vi "GetBdcst.vi"(8 "ErrorArray":errorcluster[](array[cluster]), 10 "BdcstInfo":variant, 11 "TestBase.lvclass":refnum<class "TestBase.lvclass">) -> (0 "ErrorArray":errorcluster[](array[cluster]), 3 "TestBase.lvclass":refnum<class "TestBase.lvclass">)   [LabVIEW 2014, in "TestBase.lvclass"]
uses:
  TestBase.lvclass
  TypeDefs/BdcstInfo.ctl
  TestBase.lvclass/TestBase.ctl
  WfrmGenerator/WfrmModule/Protected/Broadcasts/clBroadcastEvents.ctl
  WfrmGenerator/WfrmModule/Protected/clEventType.ctl
  Sampler/SamplerModule/Protected/Broadcasts/clBroadcastEvents.ctl
  Sampler/SamplerModule/Protected/clEventType.ctl
  FunctionGenerator/FGenModule/Protected/Broadcasts/clBroadcastEvents.ctl
  FunctionGenerator/FGenModule/Protected/clEventType.ctl
  Sync/SyncModule/Protected/Broadcasts/clBroadcastEvents.ctl
  Sync/SyncModule/Protected/clEventType.ctl
  Accessors/Read ErrorSeverity.vi
  <vilib>/Utility/error.llb/Error Cluster From Error Code.vi
  <vilib>/ErrorRing/Error Ring.xnode
  <userlib>/NIST/NISTErrorLib/NISTErrorLib.lvlib
  WfrmGenerator/WfrmModule/WfrmModule.lvlib
  Sync/SyncModule/SyncModule.lvlib
  Sampler/SamplerModule/SamplerModule.lvlib
  FunctionGenerator/FGenModule/FGenModule.lvlib
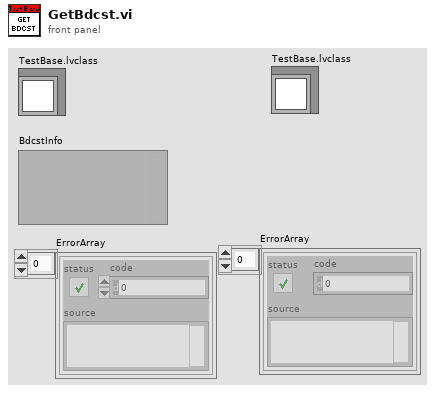
[diagram p1: front panel]
types:
  T1 = typedef "TestBase.lvclass/BdcstInfo.ctl" = cluster{"ModuleID":i32, "ModuleType":enum16{"Wfrm", "FGen", "Sampler", "Sync", "Analysis", "Sensor"}, "UserEvtRef":variant, "ScriptCmd":string}
  T2 = enum16{"Wfrm", "FGen", "Sampler", "Sync", "Analysis", "Sensor"}
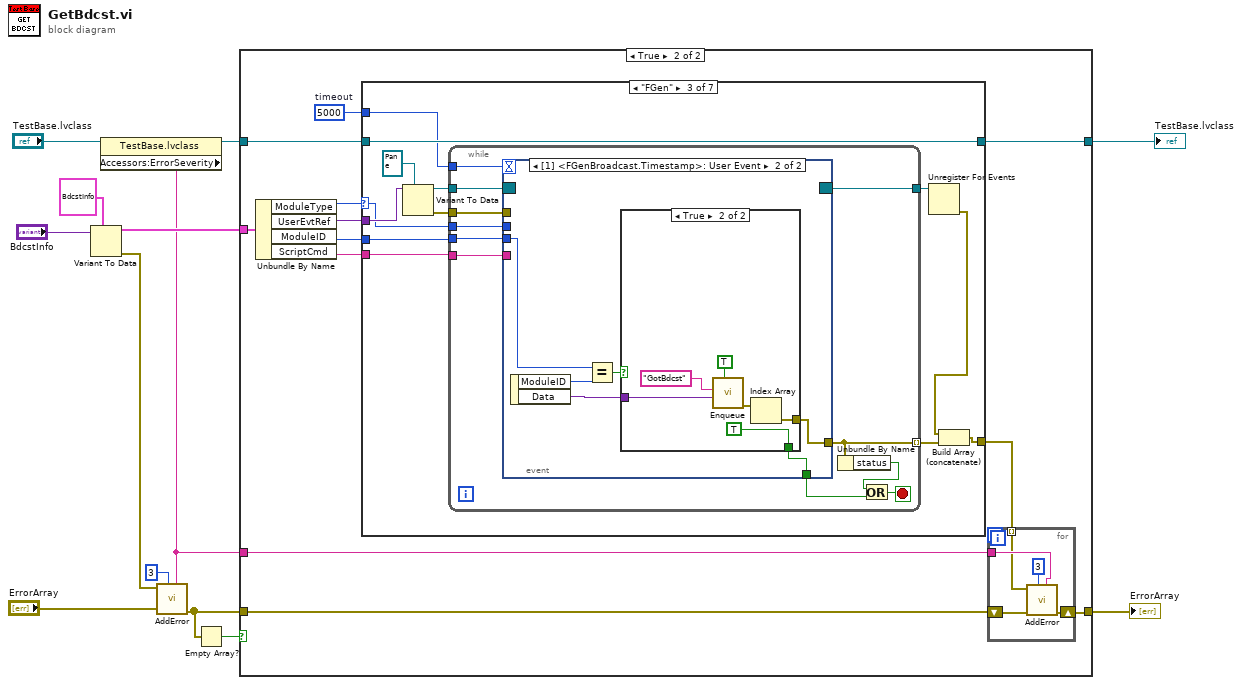
[diagram p0: block diagram]
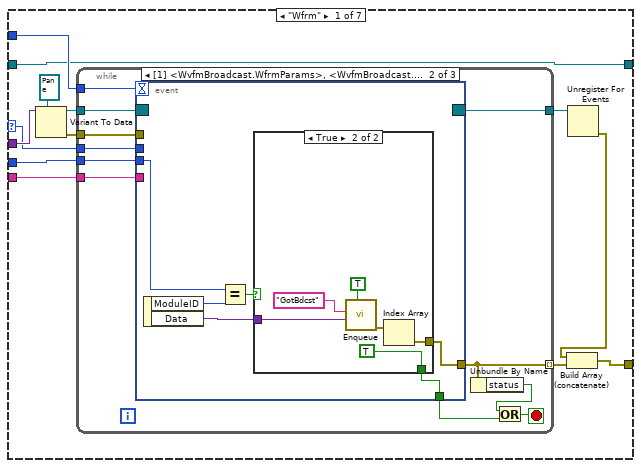
[diagram p3: hidden frame]
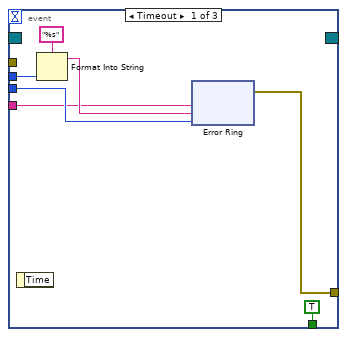
[diagram p4: hidden frame]
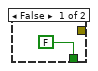
[diagram p5: hidden frame]
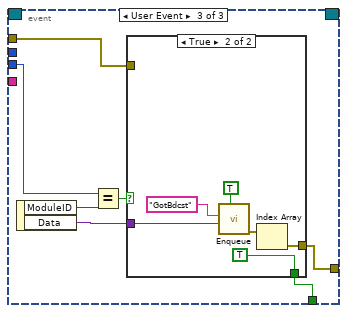
[diagram p6: hidden frame]
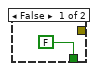
[diagram p7: hidden frame]
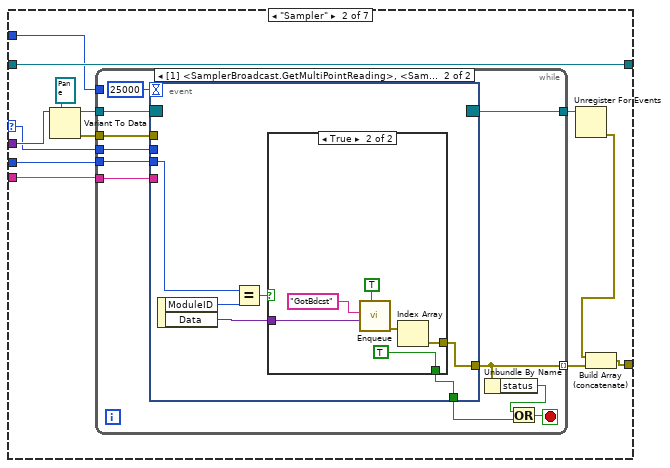
[diagram p8: hidden frame]
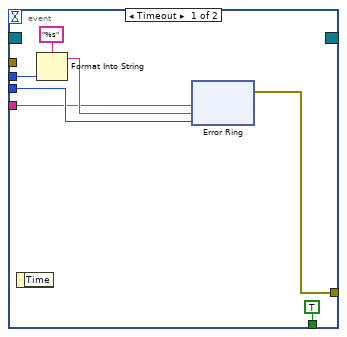
[diagram p9: hidden frame]
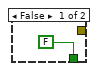
[diagram p10: hidden frame]
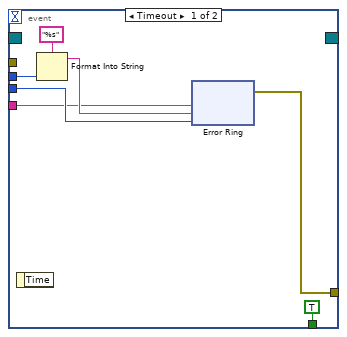
[diagram p11: hidden frame]
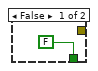
[diagram p12: hidden frame]
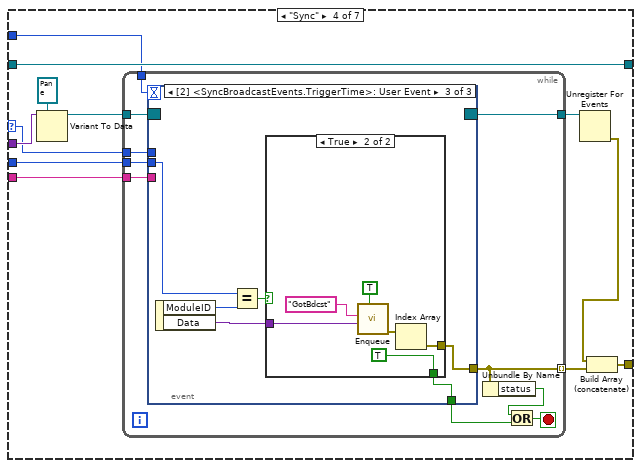
[diagram p13: hidden frame]
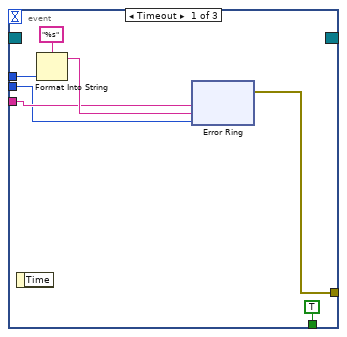
[diagram p14: hidden frame]
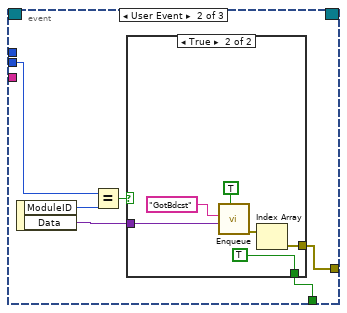
[diagram p15: hidden frame]
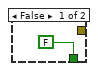
[diagram p16: hidden frame]
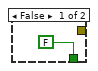
[diagram p17: hidden frame]
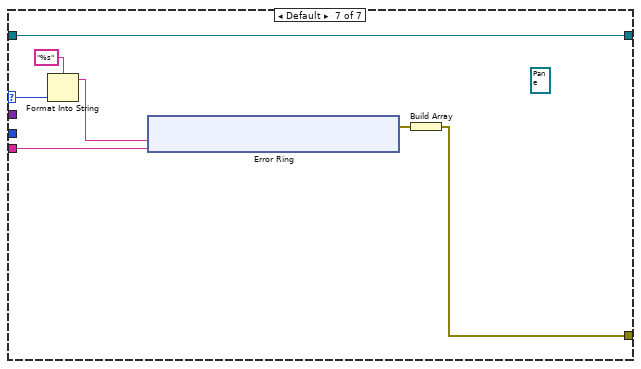
[diagram p20: hidden frame]
diagram:
  n1 = Variant To Data(type=T1 {"ModuleID"=0, "ModuleType"=enum."Wfrm", "UserEvtRef"=variant, "ScriptCmd"=""} ("BdcstInfo"), Variant="BdcstInfo") -> (data=w6:T1, error out=w9:errorcluster)  [unwired: 1 in]
  n2 = property class="TestBase.lvclass"(reference="TestBase.lvclass") -> (reference out=w5:refnum<class "TestBase.lvclass">, "Accessors:ErrorSeverity"=w3:string)  [unwired: 1 in, 1 out]
  n3 = call <userlib>:"AddError.vi"("Severity"=w3, "Priority"=u8 3, "ErrorArray"="ErrorArray", "error in (no error)"=w9) -> ("ErrorArray"=w4:errorcluster[])  [unwired: 6 in, 1 out]
  n4 = Empty Array?(array=w4) -> (empty?=w7:bool)
  n5 = case shown="True" w7 {
    tunnel: w6 -> [_ w27]
    tunnel: w5 -> [w15 w22]
    tunnel: w4 -> [w14 w18]
    tunnel: w3 -> [_ w17]
    tunnel: [w14 w19] -> w2
    tunnel: [w15 w21] -> w1
    frame False {
    }
    frame True {
      w20 = 5000  # timeout
      n6 = Unbundle By Name(w27) -> ("ModuleType"=w26:T2, "UserEvtRef"=w23:variant, "ModuleID"=w24:i32, "ScriptCmd"=w25:string)
      n7 = case shown="\"FGen\"" w26 {
        selector: w26 -> [w39 w106 w160 w212 _ _ w278]
        tunnel: w25 -> [w40 w111 w164 w210 _ _ w275]
        tunnel: w24 -> [w41 w110 w163 w211 _ _ _]
        tunnel: w23 -> [w45 w108 w162 w215 _ _ _]
        tunnel: [w38 w112 w165 w217 w270 w271 w274] -> w21
        tunnel: w22 -> [w38 w112 w165 w217 w270 w271 w274]
        tunnel: w20 -> [w42 w104 w158 w214 _ _ _]
        tunnel: [w35 w101 w155 w208 _ _ w272] -> w16
        frame "Wfrm" {
          n8 = Variant To Data(type=refnum<event-registration> refnum ("event registration refnum"), Variant=w45) -> (data=w43:refnum<event-registration>, error out=w33:errorcluster)  [unwired: 1 in]
          n9 = while {
            tunnel: w43 -> [w56]
            tunnel: w42 -> [w46]
            tunnel: w41 -> [w55]
            tunnel: w40 -> [w54]
            tunnel: w39 -> [w53]
            tunnel: [w48] -> w36 mode=indexing
            tunnel: [w49] -> w37
            tunnel: w33 -> [w47]
            stop <- w52 stop-if-true
            n10 = event shown="[1] <WvfmBroadcast.WfrmParams>, <WvfmBroadcast.ReadEvtConfig>: User Event" {
              selector: w56 -> [_ _ _]
              dyn-events: [_ _ _] -> w49
              timeout: w46 -> [_ _ _]
              tunnel: w55 -> [w61 w77 w91]
              tunnel: w54 -> [w59 _ _]
              tunnel: w53 -> [w63 _ _]
              tunnel: [w58 w74 w88] -> w48
              tunnel: [TRUE w73 w87] -> w50
              tunnel: w47 -> [_ _ w86]
              event Timeout {
                n11 = event-data() -> ()  [unwired: 1 in, 1 out]
                n12 = Format Into String(format string="%s", w63) -> (resulting string=w60:string)  [unwired: 2 in, 1 out]
                n13 = xnode "Error Ring"("parameter 0"=w59, "parameter 1"=w60, "parameter 2"=w61) -> ("error out"=w58:errorcluster)
              }
              event User Event {
                n14 = event-data() -> ("ModuleID"=w78:i32, "Data"=w75:variant)  [unwired: 1 in]
                n15 = Equal?(x=w77, y=w78) -> (x = y?=w76:bool)
                n16 = case shown="True" w76 {
                  tunnel: w75 -> [_ w84]
                  tunnel: [_ w81] -> w74
                  tunnel: [FALSE TRUE] -> w73
                  frame False {
                  }
                  frame True {
                    n17 = call "Enqueue.vi"("Priority(?) (f)"=TRUE, "Data"=w84, "Message"="GotBdcst") -> ("ErrorArray"=w82:errorcluster[])  [unwired: 8 in]
                    n18 = Index Array(array=w82) -> (element=w81:errorcluster)  [unwired: 1 in]
                  }
                }
              }
              event User Event {
                n19 = event-data() -> ("ModuleID"=w92:i32, "Data"=w89:variant)  [unwired: 1 in]
                n20 = Equal?(x=w91, y=w92) -> (x = y?=w90:bool)
                n21 = case shown="True" w90 {
                  tunnel: w89 -> [_ w98]
                  tunnel: [_ w95] -> w88
                  tunnel: [FALSE TRUE] -> w87
                  tunnel: w86 -> [_ _]
                  frame False {
                  }
                  frame True {
                    n22 = call "Enqueue.vi"("Priority(?) (f)"=TRUE, "Data"=w98, "Message"="GotBdcst") -> ("ErrorArray"=w96:errorcluster[])  [unwired: 8 in]
                    n23 = Index Array(array=w96) -> (element=w95:errorcluster)  [unwired: 1 in]
                  }
                }
              }
            }
            n24 = Unbundle By Name(w48) -> ("status"=w51:bool)
            n25 = Or(x=w51, y=w50) -> (x .or. y?=w52:bool)
          }
          n26 = Unregister For Events(event registration refnum=w37) -> (error out=w34:errorcluster)  [unwired: 1 in]
          n27 = Build Array (concatenate)(w34, w36) -> (w35:errorcluster[])
        }
        frame "Sampler" {
          n28 = Variant To Data(type=refnum<event-registration> refnum ("Event Registration Refnum"), Variant=w108) -> (data=w105:refnum<event-registration>, error out=w107:errorcluster)  [unwired: 1 in]
          n29 = while {
            tunnel: w105 -> [w123]
            tunnel: w104 -> [_]
            tunnel: w110 -> [w122]
            tunnel: w111 -> [w121]
            tunnel: w106 -> [w120]
            tunnel: [w115] -> w102 mode=indexing
            tunnel: [w116] -> w103
            tunnel: w107 -> [w114]
            stop <- w119 stop-if-true
            n30 = event shown="[1] <SamplerBroadcast.GetMultiPointReading>, <SamplerBroadcast.GetReading>: User Event" {
              selector: w123 -> [_ _]
              dyn-events: [_ _] -> w116
              timeout: 25000 -> [_ _]
              tunnel: w122 -> [w128 w144]
              tunnel: w121 -> [w126 _]
              tunnel: w120 -> [w130 _]
              tunnel: [w125 w141] -> w115
              tunnel: [TRUE w140] -> w117
              tunnel: w114 -> [_ _]
              event Timeout {
                n31 = event-data() -> ()  [unwired: 1 in, 1 out]
                n32 = Format Into String(format string="%s", w130) -> (resulting string=w127:string)  [unwired: 2 in, 1 out]
                n33 = xnode "Error Ring"("parameter 0"=w126, "parameter 1"=w127, "parameter 2"=w128) -> ("error out"=w125:errorcluster)
              }
              event User Event {
                n34 = event-data() -> ("ModuleID"=w145:i32, "Data"=w142:variant)  [unwired: 1 in]
                n35 = Equal?(x=w144, y=w145) -> (x = y?=w143:bool)
                n36 = case shown="True" w143 {
                  tunnel: w142 -> [_ w151]
                  tunnel: [_ w148] -> w141
                  tunnel: [FALSE TRUE] -> w140
                  frame False {
                  }
                  frame True {
                    n37 = call "Enqueue.vi"("Priority(?) (f)"=TRUE, "Data"=w151, "Message"="GotBdcst") -> ("ErrorArray"=w149:errorcluster[])  [unwired: 8 in]
                    n38 = Index Array(array=w149) -> (element=w148:errorcluster)  [unwired: 1 in]
                  }
                }
              }
            }
            n39 = Unbundle By Name(w115) -> ("status"=w118:bool)
            n40 = Or(x=w118, y=w117) -> (x .or. y?=w119:bool)
          }
          n41 = Unregister For Events(event registration refnum=w103) -> (error out=w100:errorcluster)  [unwired: 1 in]
          n42 = Build Array (concatenate)(w100, w102) -> (w101:errorcluster[])
        }
        frame "FGen" {
          n43 = Variant To Data(type=refnum<event-registration> refnum ("event registration refnum"), Variant=w162) -> (data=w159:refnum<event-registration>, error out=w161:errorcluster)  [unwired: 1 in]
          n44 = while {
            tunnel: w159 -> [w176]
            tunnel: w158 -> [w166]
            tunnel: w163 -> [w175]
            tunnel: w164 -> [w174]
            tunnel: w160 -> [w173]
            tunnel: [w168] -> w156 mode=indexing
            tunnel: [w169] -> w157
            tunnel: w161 -> [w167]
            stop <- w172 stop-if-true
            n45 = event shown="[1] <FGenBroadcast.Timestamp>: User Event" {
              selector: w176 -> [_ _]
              dyn-events: [_ _] -> w169
              timeout: w166 -> [_ _]
              tunnel: w175 -> [w181 w197]
              tunnel: w174 -> [w179 _]
              tunnel: w173 -> [w183 _]
              tunnel: [w178 w194] -> w168
              tunnel: [TRUE w193] -> w170
              tunnel: w167 -> [_ _]
              event Timeout {
                n46 = event-data() -> ()  [unwired: 1 in, 1 out]
                n47 = Format Into String(format string="%s", w183) -> (resulting string=w180:string)  [unwired: 2 in, 1 out]
                n48 = xnode "Error Ring"("parameter 0"=w179, "parameter 1"=w180, "parameter 2"=w181) -> ("error out"=w178:errorcluster)
              }
              event User Event {
                n49 = event-data() -> ("ModuleID"=w198:i32, "Data"=w195:variant)  [unwired: 1 in]
                n50 = Equal?(x=w197, y=w198) -> (x = y?=w196:bool)
                n51 = case shown="True" w196 {
                  tunnel: w195 -> [_ w204]
                  tunnel: [_ w201] -> w194
                  tunnel: [FALSE TRUE] -> w193
                  frame False {
                  }
                  frame True {
                    n52 = call "Enqueue.vi"("Priority(?) (f)"=TRUE, "Data"=w204, "Message"="GotBdcst") -> ("ErrorArray"=w202:errorcluster[])  [unwired: 8 in]
                    n53 = Index Array(array=w202) -> (element=w201:errorcluster)  [unwired: 1 in]
                  }
                }
              }
            }
            n54 = Unbundle By Name(w168) -> ("status"=w171:bool)
            n55 = Or(x=w171, y=w170) -> (x .or. y?=w172:bool)
          }
          n56 = Unregister For Events(event registration refnum=w157) -> (error out=w154:errorcluster)  [unwired: 1 in]
          n57 = Build Array (concatenate)(w154, w156) -> (w155:errorcluster[])
        }
        frame "Sync" {
          n58 = Variant To Data(type=refnum<event-registration> refnum ("Event Registration Refnum"), Variant=w215) -> (data=w213:refnum<event-registration>)  [unwired: 1 in, 1 out]
          n59 = while {
            tunnel: [w223] -> w207 mode=indexing
            tunnel: [w224] -> w209
            tunnel: w214 -> [w222]
            tunnel: w213 -> [w221]
            tunnel: w212 -> [w220]
            tunnel: w211 -> [w219]
            tunnel: w210 -> [w218]
            stop <- w227 stop-if-true
            n60 = event shown="[2] <SyncBroadcastEvents.TriggerTime>: User Event" {
              selector: w221 -> [_ _ _]
              dyn-events: [_ _ _] -> w224
              timeout: w222 -> [_ _ _]
              tunnel: [w232 w246 w259] -> w223
              tunnel: [TRUE w245 w258] -> w225
              tunnel: w220 -> [w230 _ _]
              tunnel: w219 -> [w228 w244 w257]
              tunnel: w218 -> [w229 _ _]
              event Timeout {
                n61 = event-data() -> ()  [unwired: 1 in, 1 out]
                n62 = Format Into String(format string="%s", w230) -> (resulting string=w233:string)  [unwired: 2 in, 1 out]
                n63 = xnode "Error Ring"("parameter 0"=w229, "parameter 1"=w233, "parameter 2"=w228) -> ("error out"=w232:errorcluster)
              }
              event User Event {
                n64 = event-data() -> ("ModuleID"=w249:i32, "Data"=w247:variant)  [unwired: 1 in]
                n65 = Equal?(x=w244, y=w249) -> (x = y?=w248:bool)
                n66 = case shown="True" w248 {
                  tunnel: w247 -> [_ w255]
                  tunnel: [_ w252] -> w246
                  tunnel: [FALSE TRUE] -> w245
                  frame False {
                  }
                  frame True {
                    n67 = call "Enqueue.vi"("Priority(?) (f)"=TRUE, "Data"=w255, "Message"="GotBdcst") -> ("ErrorArray"=w253:errorcluster[])  [unwired: 8 in]
                    n68 = Index Array(array=w253) -> (element=w252:errorcluster)  [unwired: 1 in]
                  }
                }
              }
              event User Event {
                n69 = event-data() -> ("ModuleID"=w262:i32, "Data"=w260:variant)  [unwired: 1 in]
                n70 = Equal?(x=w257, y=w262) -> (x = y?=w261:bool)
                n71 = case shown="True" w261 {
                  tunnel: w260 -> [_ w268]
                  tunnel: [_ w265] -> w259
                  tunnel: [FALSE TRUE] -> w258
                  frame False {
                  }
                  frame True {
                    n72 = call "Enqueue.vi"("Priority(?) (f)"=TRUE, "Data"=w268, "Message"="GotBdcst") -> ("ErrorArray"=w266:errorcluster[])  [unwired: 8 in]
                    n73 = Index Array(array=w266) -> (element=w265:errorcluster)  [unwired: 1 in]
                  }
                }
              }
            }
            n74 = Unbundle By Name(w223) -> ("status"=w226:bool)
            n75 = Or(x=w226, y=w225) -> (x .or. y?=w227:bool)
          }
          n76 = Unregister For Events(event registration refnum=w209) -> (error out=w206:errorcluster)  [unwired: 1 in]
          n77 = Build Array (concatenate)(w206, w207) -> (w208:errorcluster[])
        }
        frame "Analysis" {
        }
        frame "Sensor" {
        }
        frame Default {
          (unwired) refnum<event-registration> refnum ("event registration refnum")
          n78 = Format Into String(format string="%s", w278) -> (resulting string=w276:string)  [unwired: 2 in, 1 out]
          n79 = xnode "Error Ring"("parameter 0"=w276, "parameter 1"=w275) -> ("error out"=w273:errorcluster)
          n80 = Build Array(w273) -> (w272:errorcluster[])
        }
      }
      n81 = for {
        shift-right: [w31] -> w19
        shift-left: w18 -> [w30]
        tunnel: w17 -> [w29]
        tunnel: w16 -> [w28] mode=indexing
        n82 = call <userlib>:"AddError.vi"("Severity"=w29, "Priority"=u8 3, "ErrorArray"=w30, "error in (no error)"=w28) -> ("ErrorArray"=w31:errorcluster[])  [unwired: 6 in, 1 out]
      }
    }
  }
  "TestBase.lvclass" <- w1
  "ErrorArray" <- w2
